vi "SC TCP Get Duration Command.vi"(8 "error in":errorcluster, 10 "timeout (10000 ms)":i32=10000, 11 "TCP Network Connection in":refnum<k5>) -> (0 "error out":errorcluster, 3 "Duration":dbl)   [LabVIEW 2018]
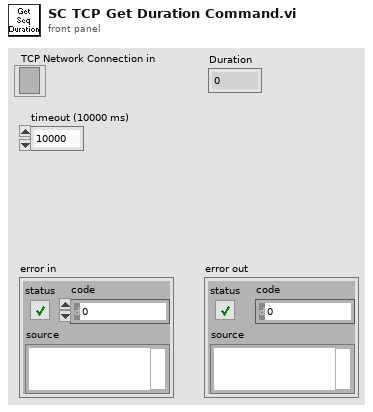
[diagram p1: front panel]
types:
  T1 = cluster{"cmdCompleted":bool, "returnType":string, "errorType":string, "errorDescription":string, "originalCommand":string, "resolvedCommand":string}
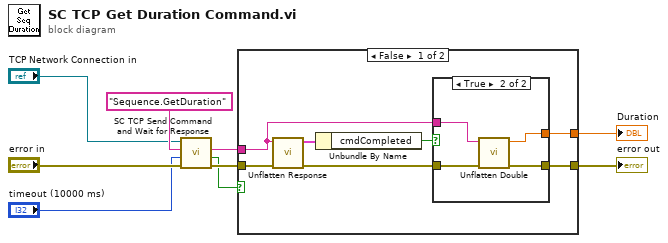
[diagram p0: block diagram]
diagram:
  n1 = call "SC TCP Send Command and Wait for Response.vi"("error in (no error)"="error in", "timeout (10000 ms)"="timeout (10000 ms)", "Command"="Sequence.GetDuration", "TCP Network Connection in"="TCP Network Connection in") -> ("error out"=w8:errorcluster, "Timed Out"=w3:bool, "Response"=w1:string)  [unwired: 4 in, 1 out]
  n2 = case shown="False" w3 {
    tunnel: [w16 w22] -> w9
    tunnel: [w15 _] -> w2
    tunnel: w1 -> [w13 _]
    tunnel: w8 -> [w11 w22]
    frame False {
      n3 = call "Unflatten Response.vi"("error in"=w11, "Response JSON"=w13) -> ("error out"=w12:errorcluster, "Response Details"=w10:T1)  [unwired: 8 in]
      n4 = Unbundle By Name(w10) -> ("cmdCompleted"=w14:bool)
      n5 = case shown="True" w14 {
        tunnel: w12 -> [w17 w21]
        tunnel: w13 -> [_ w20]
        tunnel: [_ w19] -> w15
        tunnel: [w17 w18] -> w16
        frame False {
        }
        frame True {
          n6 = call "Unflatten Double.vi"("error in"=w21, "Response JSON"=w20) -> ("error out"=w18:errorcluster, "Return Data"=w19:dbl)  [unwired: 7 in, 1 out]
        }
      }
    }
    frame True {
    }
  }
  "error out" <- w9
  "Duration" <- w2
